vi "XYStage.KIM101.GetPrivateEvents.vi"(8 "error in (no error)":errorcluster, 11 "XYStage.KIM101 in":refnum<class "XYStage.KIM101.lvclass">) -> (0 "error out":errorcluster, 2 "Private Events":T1, 3 "XYStage.KIM101 out":refnum<class "XYStage.KIM101.lvclass">)   [LabVIEW 2017, in "XYStage.KIM101.lvclass"]
uses:
  XYStage.KIM101.lvclass
  Typedefs/PrivateEvents--Cluster.ctl
  Typedefs/PrivateEvents--XYStage.KIM101.MoveAbsolute (counts).ctl
  XYStage/Typedefs/Coordinates.Counts--Cluster.ctl
  XYStage.KIM101.lvclass/XYStage.KIM101.ctl
  XYStage/XYStage.lvclass
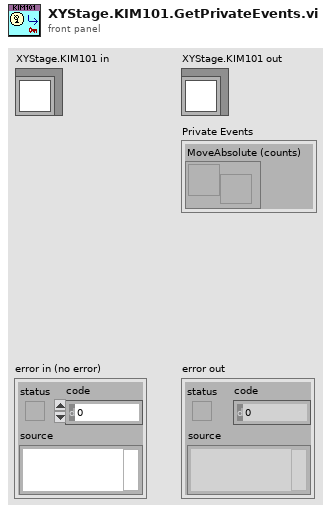
[diagram p1: front panel]
types:
  T1 = typedef "XYStage.KIM101.lvclass/PrivateEvents--Cluster.ctl" = cluster{"MoveAbsolute (counts)":refnum<user-event>}
  T2 = typedef "XYStage.KIM101.lvclass/PrivateData--Ref.ctl" = refnum<data-value>
  T3 = typedef "XYStage.KIM101.lvclass/PrivateData--Cluster.ctl" = cluster{"Resource":T4, "Private Events":T1}
  T4 = typedef "XYStage.KIM101.lvclass/Resource--Cluster.ctl" = cluster{"KCubeInertialMotorControl":refnum<k24>, "Device":refnum<k24>, "X Axis Channel":i32, "Y Axis Channel":i32}
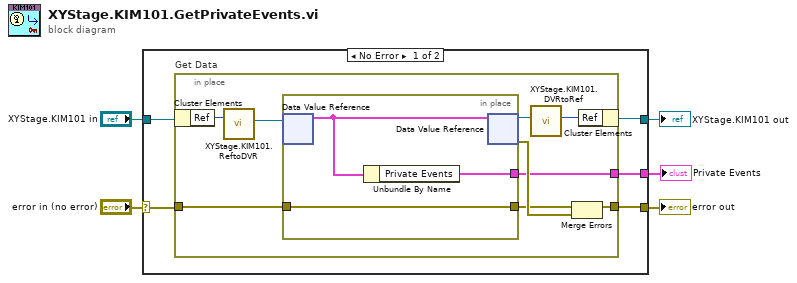
[diagram p0: block diagram]
diagram:
  n1 = case shown="No Error" "error in (no error)" {
    selector: "error in (no error)" -> [w8 w24]
    tunnel: [w7 w24] -> w4
    tunnel: [w9 w23] -> w2
    tunnel: "XYStage.KIM101 in" -> [w10 w23]
    tunnel: [w6 _] -> w1
    frame No Error {
      n2 = in-place "Get Data" {
        in-place-border: w8 -> [w19]
        in-place-border: [w16] -> w7
        in-place-border: [w15] -> w6
        n3 = in-place-cluster #1(w10) -> ("Ref"=w14:u32)
        n4 = call "XYStage.KIM101.ReftoDVR.vi"("Ref"=w14) -> ("Ref"=w13:T2)  [unwired: 10 in]
        n5 = in-place {
          in-place-border: w19 -> [w21]
          in-place-border: [w21] -> w17
          in-place-border: [w20] -> w15
          n6 = in-place-dvr #2(w13) -> (w22:T3)  [unwired: 1 out]
          n7 = Unbundle By Name(w22) -> ("Private Events"=w20:T1)
          n8 = in-place-dvr #2(w22) -> (w11:T2, w18:errorcluster)
        }
        n9 = call "XYStage.KIM101.DVRtoRef.vi"("Ref"=w11) -> ("Ref"=w12:u32)  [unwired: 10 in]
        n10 = Merge Errors(w17, w18) -> (w16:errorcluster)
        n11 = in-place-cluster #1("Ref"=w12) -> (w9:refnum<class "XYStage.KIM101.lvclass">)
      }
    }
    frame Error {
    }
  }
  "error out" <- w4
  "XYStage.KIM101 out" <- w2
  "Private Events" <- w1
